vi "Estop_test.vi"() -> ()   [LabVIEW 2021]
uses:
  Classes/Controller/Controller.lvclass
  Classes/Controller/Motion/Motion.lvclass
panel:
  out "error out":errorcluster
  in  "error in (no error)":errorcluster
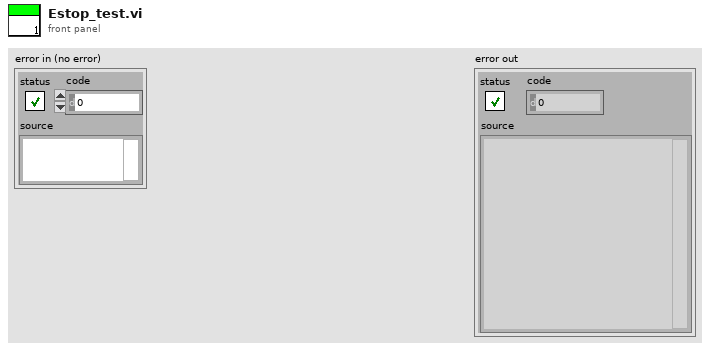
[diagram p1: front panel]
types:
  T1 = typedef "Controller.lvclass/Controllers.ctl" = cluster{"I-O.lvclass":refnum<class "I-O.lvclass">, "Gantry":refnum<k24>, "Dispenser":refnum<visa-resource-name>}
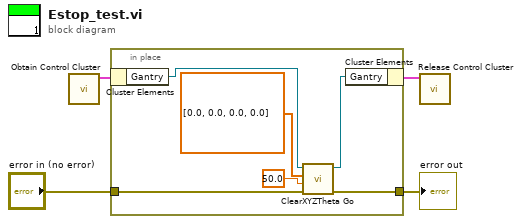
[diagram p0: block diagram]
diagram:
  n1 = call "Obtain Control Cluster.vi"() -> ("Control Out"=w4:T1)  [unwired: 10 in, 1 out]
  n2 = in-place {
    in-place-border: "error in (no error)" -> [w7]
    in-place-border: [w6] -> w2
    n3 = in-place-cluster #1(w4) -> ("Gantry"=w10:refnum<k24>)
    n4 = call "ClearXYZTheta Go.vi"("error in (no error)"=w7, "Speed"=50.0, "XYZTheta In"=dbl[] [0.0, 0.0, 0.0, 0.0], "Gantry In"=w10) -> ("error out"=w6:errorcluster, "Gantry Out"=w5:refnum<k24>)  [unwired: 5 in, 1 out]
    n5 = in-place-cluster #1("Gantry"=w5) -> (w1:T1)
  }
  "error out" <- w2
  n6 = call "Release Control Cluster.vi"("output cluster"=w1) -> ()  [unwired: 11 in]
